vi "KtFilter (SubVI).vi"(8 "N tick":u8, 9 "frq":dbl, 10 "LPF_Filter":enum16{"14 МГц", "10 МГц", "7.5 МГц", "Выкл."}(ring), 11 "Array":cluster{"Frq":dbl[], "Kt":dbl[]}[](array[cluster])) -> (3 "Numeric":dbl)   [LabVIEW 2017]
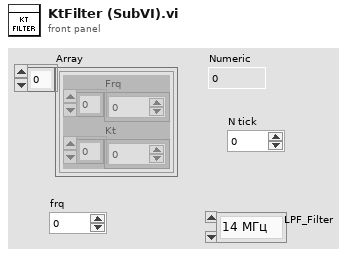
[diagram p1: front panel]
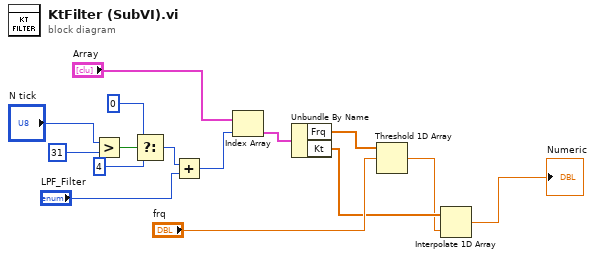
[diagram p0: block diagram]
diagram:
  n1 = Greater?(x="N tick", y=u8 31) -> (0:w6:bool)
  n2 = Select(t=0, s=w6, f=4) -> (s? t:f=w3:i32)
  n3 = Add(x=w3, y="LPF_Filter") -> (x+y=w1:i32)
  n4 = Index Array(array="Array", index=w1) -> (element=w12:cluster{"Frq":dbl[], "Kt":dbl[]})
  n5 = Unbundle By Name(w12) -> ("Frq"=w13:dbl[], "Kt"=w14:dbl[])
  n6 = Threshold 1D Array(2:"frq", 3:w13) -> (0:w9:dbl)  [unwired: 1 in]
  n7 = Interpolate 1D Array(1:w9, 2:w14) -> (0:→"Numeric":dbl)
